vi "New AS-File.vi"(7 "Data Cluster In":T1, 8 "error in":errorcluster) -> (0 "error out":errorcluster, 2 "cancelled":bool, 5 "Data Cluster Out":T1)   [LabVIEW 2021, in "AS-Configuration.lvlib"]
uses:
  AS-Configuration.lvlib
  Module Data--cluster.ctl
  Configuration/DO Channel's.ctl
  Host-Control's/DTT Test folder Name's.ctl
  Configuration/All Interface Data.ctl
  Configuration/Analog Input Single Channel Data--Cluster.ctl
  Configuration/Config-Channel Type.ctl
  Configuration/Channel Sub-Type.ctl
  Analog Output/Controls/AO Timing Cluster.ctl
  Configuration/Configuration.lvlib
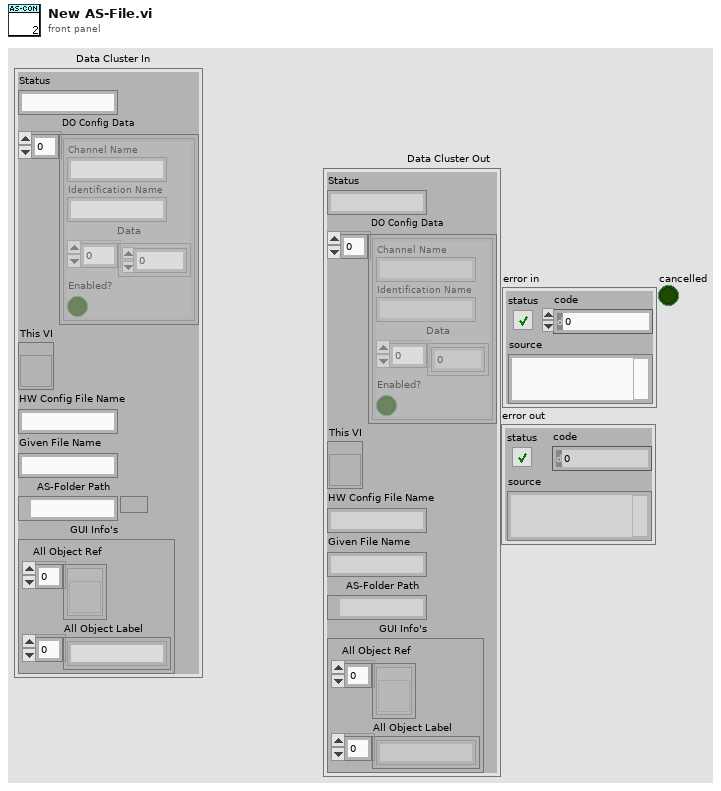
[diagram p1: front panel]
types:
  T1 = typedef "AS-Configuration.lvlib/Module Data--cluster.ctl" = cluster{"Status":string, "DO-DI Channel's":T2, "This VI":refnum<vi>, "HW Config File Name":string, "Given File Name":string, "AS-Folder Path":path, "GUI Info's":cluster{"All Object Ref":refnum<vi>[], "All Object Label":string[]}}
  T2 = typedef "Configuration.lvlib/DO Channel's.ctl" = cluster{"Channel Name":string, "Identification Name":string, "Data":u8[], "Enabled?":bool}[]
  T3 = typedef "DTT Test folder Name's.ctl" = enum16{"Event Log", "Auto Sequence Configuration", "Channel Configuration's"}
  T4 = typedef "Configuration.lvlib/All Interface Data.ctl" = cluster{"DI Config Data":T2, "DO Config Data":T2, "AI Config Data's":cluster{"Module Name":string, "AI Channel's Data":T5[], "Analog Input Timing":T8}[]}
  T5 = typedef "Configuration.lvlib/Analog Input Single Channel Data--Cluster.ctl" = cluster{"Channel Name":string, "Identification Name":string, "Channel Type":T6, "Sub-Type":T7, "Data":string, "Enabled?":bool}
  T6 = typedef "Configuration.lvlib/Config-Channel Type.ctl" = enum16{"Voltage", "Current", "Thermocouple", "Acclerometer"}
  T7 = typedef "Configuration.lvlib/Channel Sub-Type.ctl" = enum16{"None", "Pressure", "Force"}
  T8 = typedef "AO Timing Cluster.ctl" = cluster{"samples per channel":i32, "sample mode":i32, "Sampling Rate":dbl}
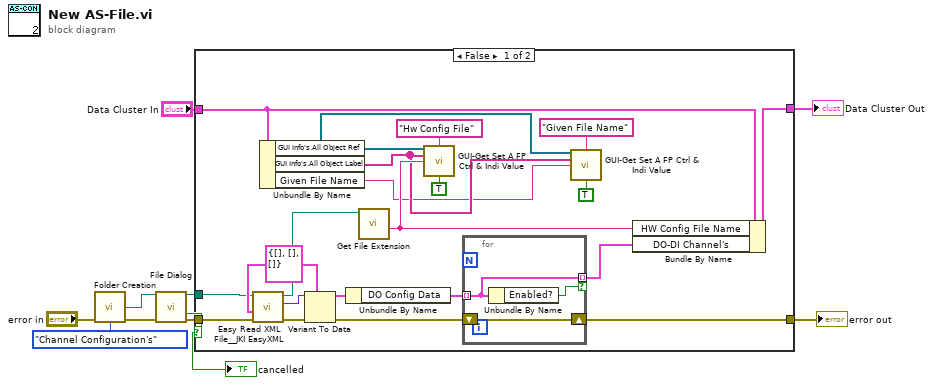
[diagram p0: block diagram]
diagram:
  n1 = call "Folder Creation.vi"("error in"="error in", "Folder Name"=DTT_Test_folder_Name's."Channel Configuration's") -> ("Selected Folder Path Out"=w6:path, "error out"=w7:errorcluster)  [unwired: 11 in, 1 out]
  n2 = call "File Dialog"("start path"=w6, "error in"=w7) -> ("selected path"=w10:path, "cancelled"=w1:bool, "error out"=w9:errorcluster)  [unwired: 10 in, 1 out]
  "cancelled" <- w1
  n3 = case shown="False" w1 {
    tunnel: w10 -> [w28 _]
    tunnel: [w20 _] -> w2
    tunnel: w9 -> [w27 _]
    tunnel: "Data Cluster In" -> [w19 w35]
    tunnel: [w21 w35] -> w3
    frame False {
      w29 = T4 {"DI Config Data"=[], "DO Config Data"=[], "AI Config Data's"=[]} ("Interface Data")
      n4 = call <vilib>:"Easy Read XML File__JKI EasyXML.vi"("error in (no error)"=w27, "LabVIEW Data (Type)"=w29, "XML File Path"=w28) -> ("error out"=w30:errorcluster, "LabVIEW Data"=w31:variant, "XML File Path (duplicate)"=w23:path)  [unwired: 6 in]
      n5 = Unbundle By Name(w19) -> ("GUI Info's.All Object Ref"=w13:refnum<vi>[], "GUI Info's.All Object Label"=w12:string[], "Given File Name"=w11:string)
      n6 = Variant To Data(error in=w30, type=w29, Variant=w31) -> (data=w24:T4, error out=w25:errorcluster)
      n7 = Unbundle By Name(w24) -> ("DO Config Data"=w26:T2)
      n8 = call <vilib>:"Get File Extension.vi"("file"=w23) -> ("filename without extension"=w16:string)  [unwired: 6 in, 4 out]
      n9 = call "GUI-Get Set A FP Ctrl & Indi Value.vi"("All Object Ref"=w13, "Label"="Hw Config File" ("Label In"), "All Object Label"=w12, "Ctrl Value In"=w16, "Set(F)"=TRUE) -> ()  [unwired: 7 in, 4 out]
      n10 = for {
        tunnel: w26 -> [w33] mode=indexing
        shift-right: [w34] -> w20
        shift-left: w25 -> [w34]
        tunnel: [w33] -> w22 mode=indexing if=w32
        n11 = Unbundle By Name(w33) -> ("Enabled?"=w32:bool)
      }
      n12 = call "GUI-Get Set A FP Ctrl & Indi Value.vi"("All Object Ref"=w13, "Label"="Given File Name" ("Label In"), "All Object Label"=w12, "Ctrl Value In"=w11, "Set(F)"=TRUE) -> ()  [unwired: 7 in, 4 out]
      n13 = Bundle By Name(cluster=w19, "HW Config File Name"=w16, "DO-DI Channel's"=w22) -> (w21:T1)
    }
    frame True {
      # "User Pressed the Cancel Button so we no need to open any file's or folder."
    }
  }
  "Data Cluster Out" <- w3
  "error out" <- w2
